vi "rotated_picture_rotate.vi"(4 "Numeric":dbl, 5 "ONE-8-bit pixmap":u8[][](array[numeric]), 6 "Seven-new element/subarray":u32, 7 "Two-Array":cdb[][](array[numeric]), 8 "Six-colors":u32[](array[numeric]), 9 "Five-Numeric 3":cdb, 10 "Four-Numeric":i32, 11 "Three-Numeric in":i32) -> (3 "new picture":picture)   [LabVIEW 2019]
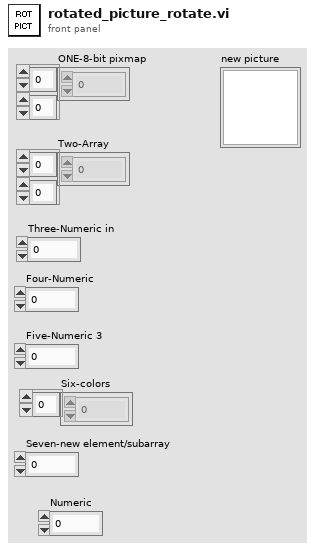
[diagram p1: front panel]
types:
  T1 = typedef "imagedata.ctl" = cluster{"image type":i32, "image depth":i32, "image":u8[], "mask":u8[], "colors":u32[], "Rectangle":cluster{"left":i16, "top":i16, "right":i16, "bottom":i16}}
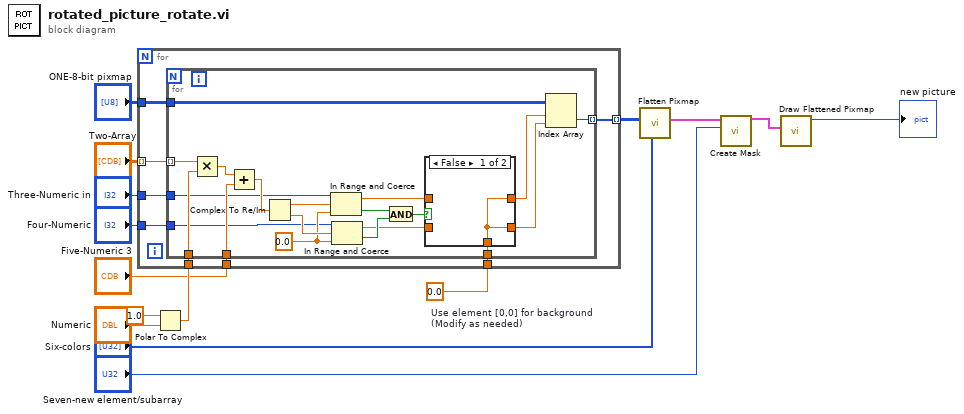
[diagram p0: block diagram]
diagram:
  w10 = 0.0  # Use element [0,0] for background (Modify as needed)
  n1 = Polar To Complex(1:"Numeric", 2:1.0 ("r")) -> (0:w11:cdb)
  n2 = for {
    tunnel: w11 -> [w23]
    tunnel: "ONE-8-bit pixmap" -> [w22]
    tunnel: "Five-Numeric 3" -> [w21]
    tunnel: "Two-Array" -> [w20] mode=indexing
    tunnel: [w19] -> w7 mode=indexing
    tunnel: w10 -> [w18]
    tunnel: "Three-Numeric in" -> [w17]
    tunnel: "Four-Numeric" -> [w16]
    n3 = for {
      tunnel: w22 -> [w43]
      tunnel: w23 -> [w38]
      tunnel: [w42] -> w19 mode=indexing
      tunnel: w21 -> [w40]
      tunnel: w20 -> [w37] mode=indexing
      tunnel: w18 -> [w24]
      tunnel: w17 -> [w32]
      tunnel: w16 -> [w31]
      w33 = 0.0 ("lower limit")
      n4 = Multiply(x=w37, y=w38) -> (x*y=w39:cdb)
      n5 = Add(x=w39, y=w40) -> (x+y=w41:cdb)
      n6 = Complex To Re/Im(x + iy=w41) -> (x=w36:dbl, y=w35:dbl)
      n7 = In Range and Coerce(upper limit=w32, x=w36, lower limit=w33) -> (coerced(x)=w27:dbl, In Range?=w34:bool)
      n8 = In Range and Coerce(upper limit=w31, x=w35, lower limit=w33) -> (coerced(x)=w25:dbl, In Range?=w30:bool)
      n9 = And(x=w34, y=w30) -> (x .and. y?=w29:bool)
      n10 = case shown="False" w29 {
        tunnel: [w44 w46] -> w28
        tunnel: w27 -> [_ w46]
        tunnel: [w44 w45] -> w26
        tunnel: w25 -> [_ w45]
        tunnel: w24 -> [w44 _]
        frame False {
        }
        frame True {
        }
      }
      n11 = Index Array(array=w43, index (row)=w28, index (col)=w26) -> (element=w42:u8)
    }
  }
  n12 = call <vilib>:"Flatten Pixmap.vi"("colors"="Six-colors", "8-bit pixmap"=w7) -> ("image data"=w13:T1)  [unwired: 9 in]
  n13 = call <vilib>:"Create Mask.vi"("Mask Color (Black)"="Seven-new element/subarray", "image data"=w13) -> ("image data"=w14:T1)  [unwired: 9 in]
  n14 = call <vilib>:"Draw Flattened Pixmap.vi"("image data"=w14) -> ("new picture"=→"new picture":picture)  [unwired: 8 in]
